vi "StopControl.vi"(8 "WindowButton":refnum<vi>, 9 "StopButton":refnum<vi>, 10 "Window mode notifier in":refnum<notifier>, 11 "Stop Notifier in":refnum<notifier>) -> ()   [LabVIEW 2015]
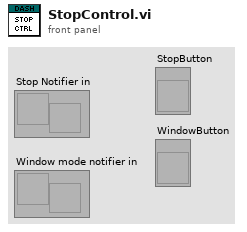
[diagram p1: front panel]
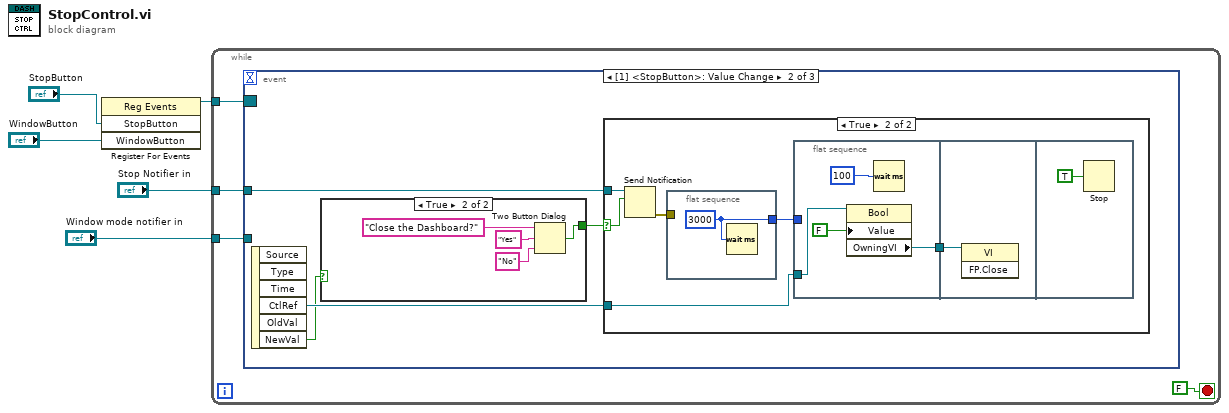
[diagram p0: block diagram]
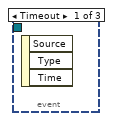
[diagram p2: hidden frame]
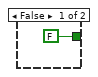
[diagram p3: hidden frame]
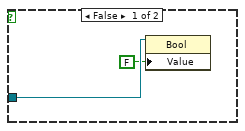
[diagram p4: hidden frame]
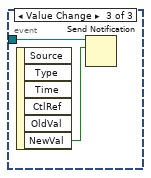
[diagram p5: hidden frame]
diagram:
  n1 = register-events("StopButton", "WindowButton") -> (reference out=w2:refnum<event-registration>)  [unwired: 2 in, 1 out]
  n2 = while {
    tunnel: "Window mode notifier in" -> [w8]
    tunnel: "Stop Notifier in" -> [w7]
    tunnel: w2 -> [w6]
    stop <- FALSE stop-if-true
    n3 = event shown="[1] <StopButton>: Value Change" {
      selector: w6 -> [_ _ _]
      dyn-events: _ -> [_ _ _]
      timeout: _ -> [_ _ _]
      tunnel: w8 -> [_ _ w35]
      tunnel: w7 -> [_ w13 _]
      event Timeout {
        n4 = event-data() -> ()  [unwired: 1 in, 3 out]
      }
      event Value Change {
        n5 = event-data() -> ("CtlRef"=w12:refnum<vi>, "NewVal"=w11:bool)  [unwired: 1 in, 4 out]
        n6 = case shown="True" w11 {
          tunnel: [FALSE ("T button?") w15] -> w10
          frame False {
          }
          frame True {
            n7 = Two Button Dialog(message="Close the Dashboard?", 1:"No" ("F button name (\"Cancel\")"), 2:"Yes" ("T button name (\"OK\")")) -> (T button?=w15:bool)
          }
        }
        n8 = case shown="True" w10 {
          selector: w10 -> [_ w21]
          tunnel: w13 -> [_ w25]
          tunnel: w12 -> [w20 w22]
          frame False {
            n9 = property class="Bool"(reference=w20, "Value"=FALSE) -> ()  [unwired: 1 in, 2 out]
          }
          frame True {
            n10 = Send Notification(notification=w21, notifier=w25) -> (error out=w24:errorcluster)  [unwired: 1 in, 1 out]
            n11 = flat-sequence {
              tunnel: w24 -> [_]
              tunnel: [w27] -> w23
              frame #0 {
                w27 = u32 3000 ("milliseconds to wait")
                n12 = Wait (ms)(milliseconds to wait=w27) -> ()  [unwired: 1 out]
              }
            }
            n13 = flat-sequence {
              tunnel: w23 -> [_]
              tunnel: w22 -> [w30]
              tunnel: [w28] -> w26
              tunnel: w26 -> [w32]
              frame #0 {
                n14 = property class="Bool"(reference=w30, "Value"=FALSE) -> ("OwningVI"=w28:refnum<vi>)  [unwired: 1 in, 2 out]
                n15 = Wait (ms)(milliseconds to wait=u32 100) -> ()  [unwired: 1 out]
              }
              frame #1 {
                n16 = invoke class="VI" method="FP.Close"(reference=w32) -> ()  [unwired: 2 in, 3 out]
              }
              frame #2 {
                n17 = Stop(stop? (T)=TRUE) -> ()
              }
            }
          }
        }
      }
      event Value Change {
        n18 = event-data() -> ("NewVal"=w34:bool)  [unwired: 1 in, 5 out]
        n19 = Send Notification(notification=w34, notifier=w35) -> ()  [unwired: 1 in, 2 out]
      }
    }
  }
